vi "Other Status.vi"(0 "Model in":refnum<class "Model.lvclass">) -> ()   [LabVIEW 2016, in "M1M3SupportEUI_Views.lvlib"]
uses:
  M1M3SupportEUI_Views.lvlib
  Model/Model.lvclass
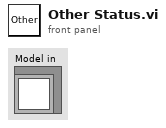
[diagram p1: front panel]
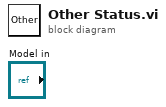
[diagram p0: block diagram]
diagram:
